vi "Clear Errors for Previous Version.vi"(8 "error in (no error)":errorcluster, 11 "code":i32) -> (0 "error out":errorcluster)   [LabVIEW 2017]
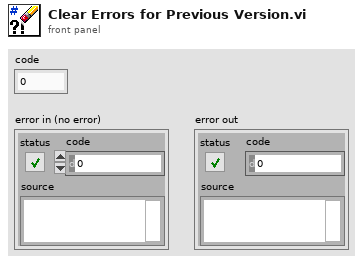
[diagram p1: front panel]
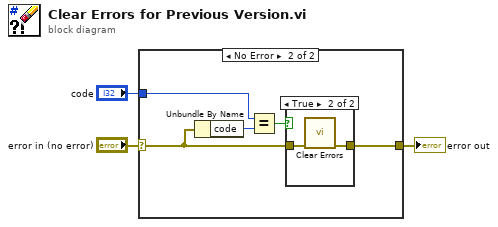
[diagram p0: block diagram]
diagram:
  n1 = case shown="No Error" "error in (no error)" {
    selector: "error in (no error)" -> [w4 w9]
    tunnel: "code" -> [_ w7]
    tunnel: [w4 w5] -> w1
    frame Error {
    }
    frame No Error {
      n2 = Unbundle By Name(w9) -> ("code"=w8:i32)
      n3 = Equal?(x=w7, y=w8) -> (x = y?=w6:bool)
      n4 = case shown="True" w6 {
        tunnel: w9 -> [w10 w12]
        tunnel: [w10 w11] -> w5
        frame False {
        }
        frame True {
          n5 = call <vilib>:"Clear Errors.vi"("error in (no error)"=w12) -> ("error out"=w11:errorcluster)  [unwired: 5 in, 1 out]
        }
      }
    }
  }
  "error out" <- w1
